vi "AcqErrorGlobalTlog.vi"() -> ()   [LabVIEW 2010]
panel:
  in  "error in (no error)":errorcluster
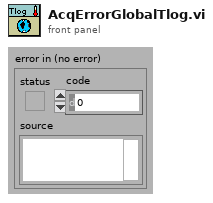
[diagram p1: front panel]
diagram:
